vi "FilterTextDeco.vi"(1 "Decos[]":refnum<vi>[](array[refnum])) -> (0 "TextDecos":refnum<vi>[](array[refnum]))   [LabVIEW 2018]
doc: "从装饰控件中过滤出文本装饰控件"
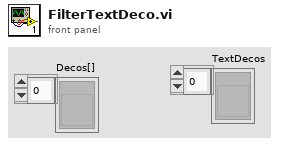
[diagram p1: front panel]
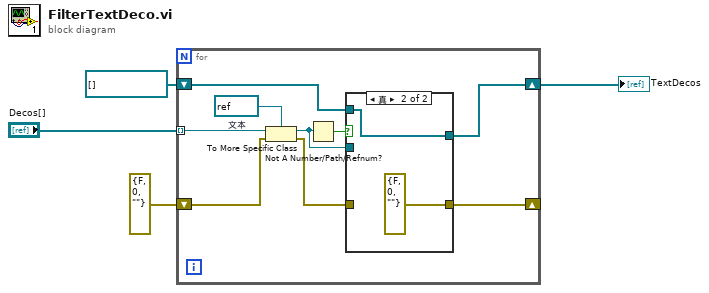
[diagram p0: block diagram]
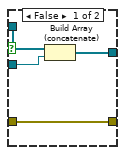
[diagram p2: hidden frame]
diagram:
  n1 = for {
    tunnel: "Decos[]" -> [w13] mode=indexing
    shift-right: [w9] -> w2
    shift-left: refnum<vi>[] [] -> [w8]
    shift-right: [w7] -> _
    shift-left: errorcluster {"status"=FALSE, "code"=0, "source"=""} ("错误常量") -> [w6]
    w12 = refnum<vi> refnum  # 文本
    n2 = To More Specific Class(target class=w12, reference=w13, error in=w6) -> (specific class reference=w10:refnum<vi>, error out=w5:errorcluster)
    n3 = Not A Number/Path/Refnum?(number/path/refnum=w10) -> (NaN/Path/Refnum?=w11:bool)
    n4 = case shown="真" w11 {
      tunnel: w10 -> [w17 _]
      tunnel: [w16 w19] -> w9
      tunnel: w8 -> [w15 w19]
      tunnel: w5 -> [w14 _]
      tunnel: [w14 errorcluster {"status"=FALSE, "code"=0, "source"=""} ("错误常量")] -> w7
      frame False {
        n5 = Build Array (concatenate)(w15, w17) -> (w16:refnum<vi>[])
      }
      frame True {
      }
    }
  }
  "TextDecos" <- w2
